vi "Control_Init_Done.vi"(8 "error in (no error)":errorcluster, 10 "Variant":variant, 11 "Camera_Scan_Controller.lvlib:Camera_Scan_Controller.lvclass":refnum<class "Camera_Scan_Controller.lvclass">) -> (0 "error out":errorcluster, 3 "Camera_Scan_Controller.lvlib:Camera_Scan_Controller.lvclass":refnum<class "Camera_Scan_Controller.lvclass">)   [LabVIEW 2023, in "Camera_Scan_Controller.lvlib" / "Camera_Scan_Controller.lvclass"]
uses:
  Camera_Scan_Controller.lvclass
  Camera_Scan_Controller.lvclass/Camera_Scan_Controller.ctl
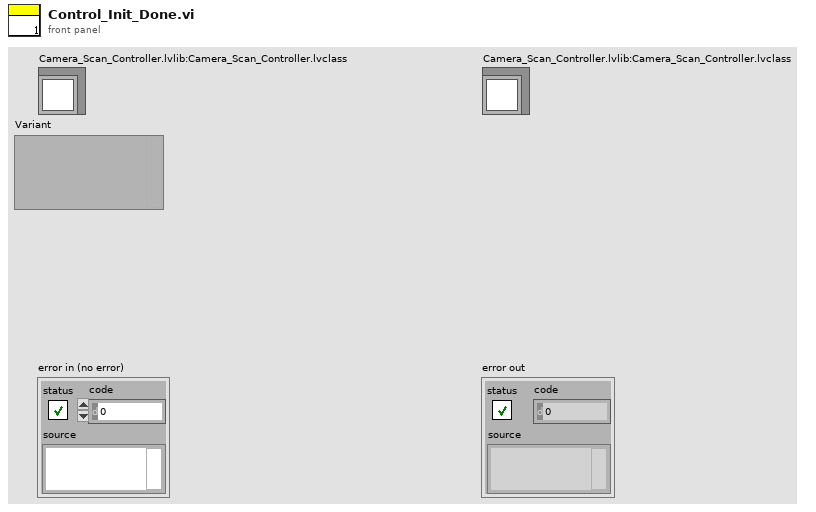
[diagram p1: front panel]
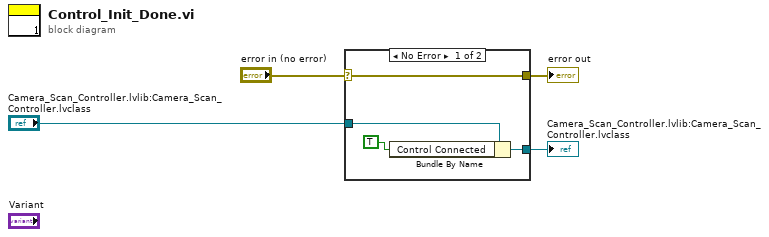
[diagram p0: block diagram]
diagram:
  n1 = case shown="No Error" "error in (no error)" {
    selector: "error in (no error)" -> [w8 w10]
    tunnel: [w8 w10] -> w3
    tunnel: [w5 w9] -> w1
    tunnel: "Camera_Scan_Controller.lvlib:Camera_Scan_Controller.lvclass" -> [w6 w9]
    frame No Error {
      n2 = Bundle By Name(cluster=w6, "Control Connected"=TRUE ("SLM Connected")) -> (w5:refnum<class "Camera_Scan_Controller.lvclass">)
    }
    frame Error {
    }
  }
  "error out" <- w3
  "Camera_Scan_Controller.lvlib:Camera_Scan_Controller.lvclass" <- w1
